vi "Enable_Relays.vi"(8 "error in (no error)":errorcluster caption="entrée d'erreur (pas d'erreur)", 11 "Class Relay_Board usb_relay_device en entrée":refnum<class "Class Relay_Board usb_Relay_device.lvclass">) -> (0 "error out":errorcluster caption="sortie d'erreur", 3 "Class Relay_Board usb_relay_device en sortie":refnum<class "Class Relay_Board usb_Relay_device.lvclass">)   [LabVIEW 2020, in "Library Instrument & Equipement.lvlib" / "Library Relay_Board.lvlib" / "Class Relay_Board usb_Relay_device.lvclass"]
uses:
  Class Relay_Board usb_Relay_device.lvclass
  C:/Users/ngarcin/OneDrive - Altyor/Standard TB/Class/Relay_Board/Relay_Board (Default)/Class Relay_Board (Default).lvclass
  Class Relay_Board usb_Relay_device.lvclass/Class Relay_Board usb_Relay_device.ctl
  Commun VI/TypeDef/Liste Error.ctl
  Commun VI/Library Commun.lvlib
  usb_relay_device/usb_relay_device.lvlib
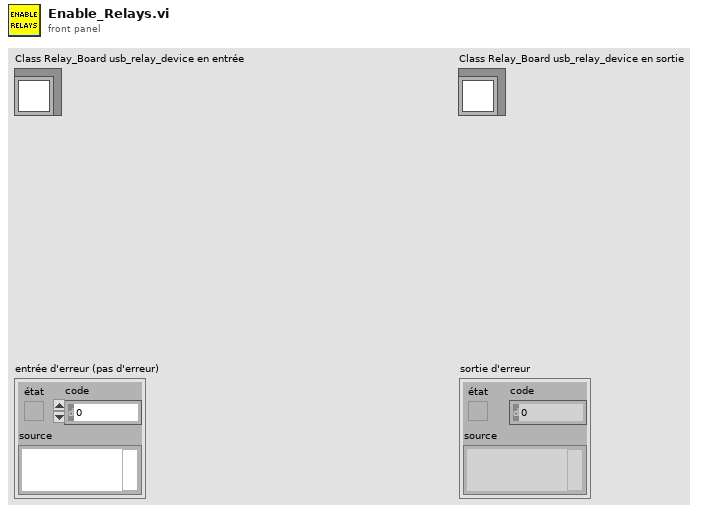
[diagram p1: front panel]
types:
  T1 = typedef "Library Commun.lvlib/Liste Error.ctl" = enum16{"Firebase Driver - Get Document", "Firebase Driver - Get Document With Where", "Firebase Driver - Delete Document", "Firebase Driver - Set Document", "Firebase Driver - Update Document", "Firebase Altyor - Search Document Bench", "Firebase Altyor - Class Not in Firebase", "Spectrum_Analyser - Timeout", "Relay Board - Qty Relay", "DIO - Pb Funtion", "Power_Supply - Peripherical not find", "Mutimeter - Peripherical not find", "Instrument - Function Not Used", "Instrument - Instrument name not specified", "Instrument - Allready Initialised", "Instrument - TimeOut", "Instrument - the instrument must be Initialise before", "Instrument - Frame Not received", "Instrument - Frame Nok", "Test - Initialise the File_for_Save", "Test - Timeout", "Test - Cmd Error", "FGV - Variable ", "BDD FireBase - Define Class", "SN - Class Not Define"}
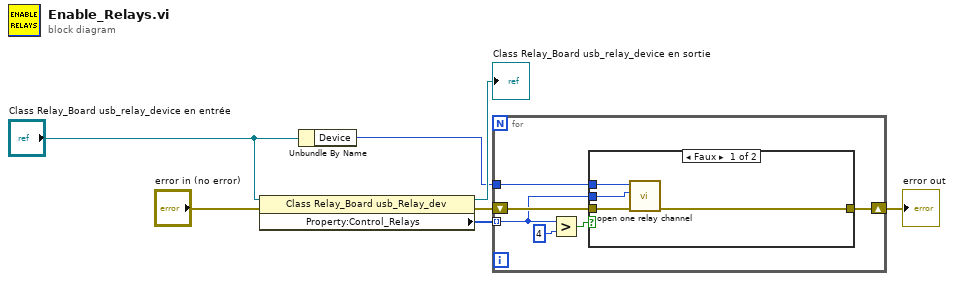
[diagram p0: block diagram]
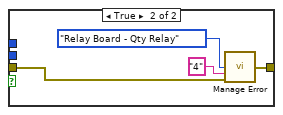
[diagram p2: hidden frame]
diagram:
  n1 = property class="Class Relay_Board usb_Relay_dev"(reference="Class Relay_Board usb_relay_device en entrée", error in="error in (no error)") -> (reference out=→"Class Relay_Board usb_relay_device en sortie":refnum<class "Class Relay_Board usb_Relay_device.lvclass">, error out=w7:errorcluster, "Property:Control_Relays"=w6:u8[])
  n2 = Unbundle By Name("Class Relay_Board usb_relay_device en entrée") -> ("Device"=w1:i32)
  n3 = for {
    shift-right: [w11] -> w3
    shift-left: w7 -> [w13]
    tunnel: w6 -> [w10] mode=indexing
    tunnel: w1 -> [w12]
    n4 = Greater?(x=w10, y=u8 4) -> (0:w8:bool)
    n5 = case shown="Faux" w8 {
      tunnel: w13 -> [w17 w18]
      tunnel: w12 -> [w14 _]
      tunnel: [w16 w20] -> w11
      tunnel: w10 -> [w15 _]
      frame False {
        n6 = call "open one relay channel.vi"("error in (no error)"=w17, "index"=w15, "hHandle"=w14) -> ("error out"=w16:errorcluster)  [unwired: 8 in]
      }
      frame True {
        n7 = call "Manage Error.vi"("Code Erreur"=Liste_Error."Relay Board - Qty Relay", "Text"="4", "error in (no error)"=w18) -> ("error out"=w20:errorcluster)  [unwired: 12 in]
      }
    }
  }
  "error out" <- w3
